vi "double_string_conversion.vi"(11 "appended array":dbl[](array[numeric])=[-2.980680317413301e-06, 3.302355013397003e-06, 2.4310694825512846e-06, -2.0001319181033614e-06, -1.511612756413447e-08, 1.943785118141561e-08, -7.187559800358143e-07, 1.071844380502973e-06, 1.9000010869058017, -1.1536739062188952e-06, 2.9999999995136135, 5.804690291396179e-10]) -> (3 "concatenated string":string)   [LabVIEW 2015]
panel:
  in  "precision (6)":i16
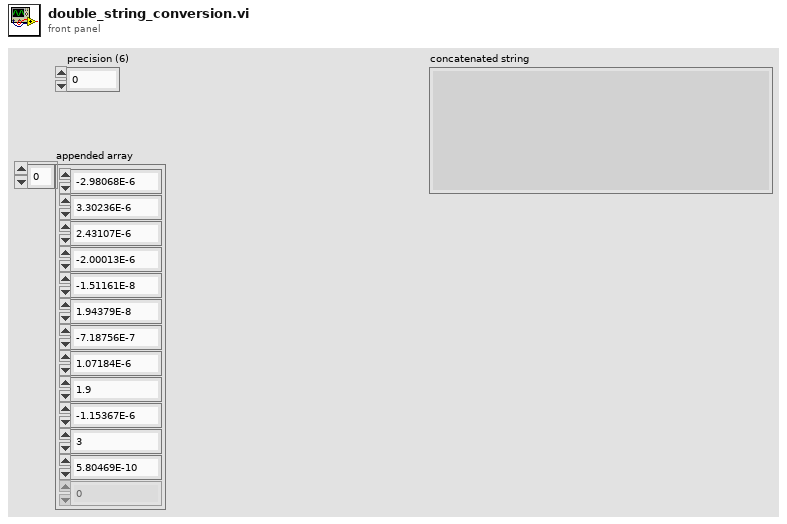
[diagram p1: front panel]
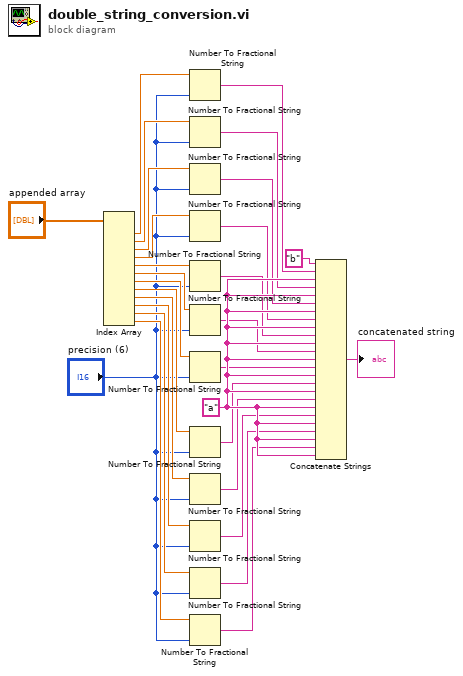
[diagram p0: block diagram]
diagram:
  w27 = "a"
  n1 = Index Array ("Index Array 6")(array="appended array") -> (element #1=w24:dbl, element #2=w22:dbl, element #3=w20:dbl, element #4=w18:dbl, element #5=w16:dbl, element #6=w14:dbl, element #7=w12:dbl, element #8=w10:dbl, element #9=w8:dbl, element #10=w6:dbl, element #11=w4:dbl, element #12=w2:dbl)  [unwired: 12 in]
  n2 = Number To Fractional String(number=w24, precision (6)="precision (6)") -> (F-format string=w25:string)  [unwired: 2 in]
  n3 = Number To Fractional String(number=w22, precision (6)="precision (6)") -> (F-format string=w23:string)  [unwired: 2 in]
  n4 = Number To Fractional String(number=w20, precision (6)="precision (6)") -> (F-format string=w21:string)  [unwired: 2 in]
  n5 = Number To Fractional String(number=w18, precision (6)="precision (6)") -> (F-format string=w19:string)  [unwired: 2 in]
  n6 = Number To Fractional String(number=w16, precision (6)="precision (6)") -> (F-format string=w17:string)  [unwired: 2 in]
  n7 = Number To Fractional String(number=w14, precision (6)="precision (6)") -> (F-format string=w15:string)  [unwired: 2 in]
  n8 = Number To Fractional String(number=w12, precision (6)="precision (6)") -> (F-format string=w13:string)  [unwired: 2 in]
  n9 = Number To Fractional String(number=w10, precision (6)="precision (6)") -> (F-format string=w11:string)  [unwired: 2 in]
  n10 = Number To Fractional String(number=w8, precision (6)="precision (6)") -> (F-format string=w9:string)  [unwired: 2 in]
  n11 = Number To Fractional String(number=w6, precision (6)="precision (6)") -> (F-format string=w7:string)  [unwired: 2 in]
  n12 = Number To Fractional String(number=w4, precision (6)="precision (6)") -> (F-format string=w5:string)  [unwired: 2 in]
  n13 = Number To Fractional String(number=w2, precision (6)="precision (6)") -> (F-format string=w3:string)  [unwired: 2 in]
  n14 = Concatenate Strings("b", w25, w27, w23, w27, w21, w27, w19, w27, w17, w27, w15, w27, w13, w27, w11, w27, w9, w27, w7, w27, w5, w27, w3, w27) -> (→"concatenated string":string)
